vi "get_Image_from_multipage_TIFF.vi"(8 "error in (no error)":errorcluster, 11 "ImageCollection in":refnum<class "ImageCollection.lvclass">) -> (0 "error out":errorcluster, 2 "image":refnum<class "Image.lvclass">, 3 "ImageCollection out":refnum<class "ImageCollection.lvclass">)   [LabVIEW 2010]
uses:
  main/dlls/saveTiffStack_v02b/tiff_manage.dll
  Image/Image/Image.lvclass
  ImageCollection.lvclass
panel:
  in  "page_nr":u32=1
  out "return type":i32
  out "compression":u32
  out "bitspersample":u32
  out "length":u32
  out "width":u32
  out "status":u16
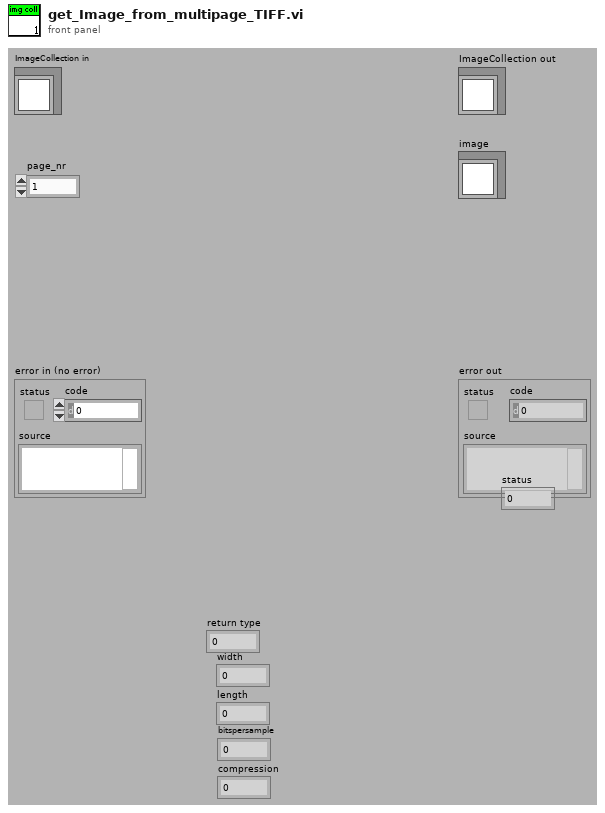
[diagram p1: front panel]
types:
  T1 = typedef "Image Type" = u32
  T2 = typedef "IMAQ Image.ctl" = refnum<image>
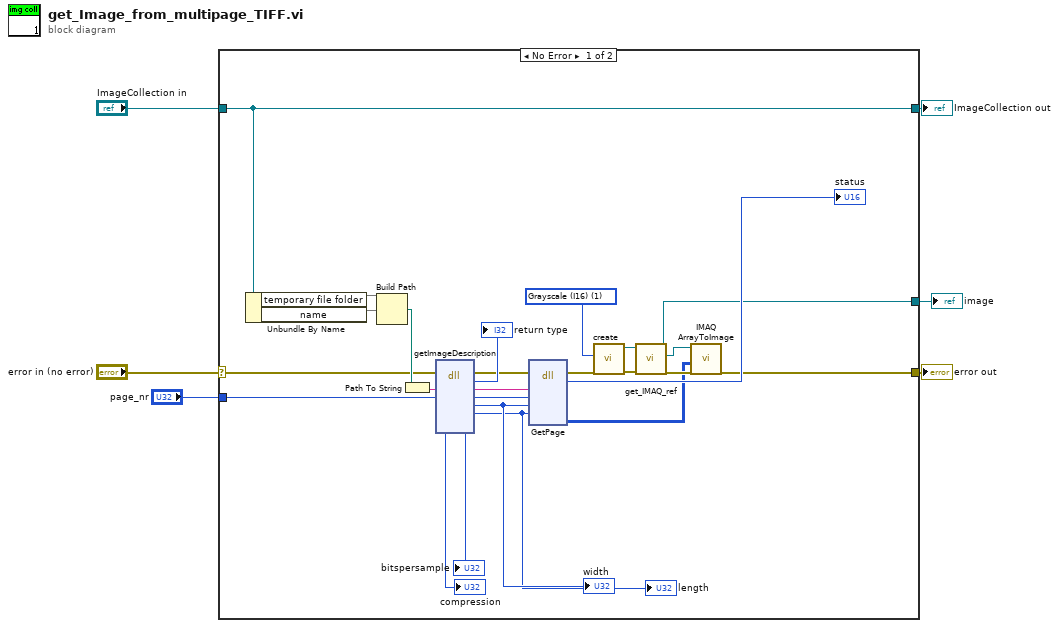
[diagram p0: block diagram]
diagram:
  n1 = case shown="No Error" "error in (no error)" {
    selector: "error in (no error)" -> [w19 w33]
    tunnel: [w13 w33] -> w5
    tunnel: [w31 w32] -> w3
    tunnel: "ImageCollection in" -> [w31 w32]
    tunnel: "page_nr" -> [w20 _]
    tunnel: [w9 _] -> w1
    frame No Error {
      w10 = T1 1 items=["Grayscale (U8)", "Grayscale (I16)", "Grayscale (SGL)", "Complex (CSG)", "RGB (U32)", "HSL (U32)", "RGB (U64)", "Grayscale (U16)"] ("Image Type")
      n2 = Unbundle By Name(w31) -> ("temporary file folder"=w30, "name"=w29)
      n3 = Build Path(base path=w30, name or relative path=w29) -> (appended path=w21:path)
      n4 = Path To String(path=w21) -> (string=w22:string)
      n5 = dll-call lib="C:/helioscan/main/dlls/saveTiffStack_v02b/tiff_manage.dll" fn="getImageDescription"(error in=w19, "path_filename"=w22, "page_nr"=w20) -> (error out=w18:errorcluster, "return value"=→"return type":i32, "path_filename"=w8:string, "page_nr"=w7:u32, "width"=w25:u32, "length"=w24:u32, "bitspersample"=→"bitspersample":u32, "compression"=→"compression":u32)  [unwired: 6 in, 1 out]
      "width" <- w25
      "length" <- w24
      n6 = dll-call lib="C:/helioscan/main/dlls/saveTiffStack_v02b/tiff_manage.dll" fn="GetPage"(error in=w18, "path_filename"=w8, "page_nr"=w7, "nrows"=w25, "ncols"=w24) -> (error out=w16:errorcluster, "return value"=→"status":u16, "in_array"=w12:u16[][])  [unwired: 7 in, 1 out]
      n7 = call "create.vi"("error in (no error)"=w16, "Image Type"=w10) -> ("error out"=w17:errorcluster, "Image out"=w15:refnum<class "Image.lvclass">)  [unwired: 8 in]
      n8 = call-dynamic "get_IMAQ_ref.vi"("error in (no error)"=w17, "Image.lvclass in"=w15) -> ("error out"=w14:errorcluster, "Image"=w11:T2, "Image.lvclass out"=w9:refnum<class "Image.lvclass">)  [unwired: 5 in, 2 out]
      n9 = call "IMAQ ArrayToImage"("error in (no error)"=w14, "Image Pixels (I16)"=w12, "Image"=w11) -> ("error out"=w13:errorcluster)  [unwired: 7 in, 1 out]
    }
    frame Error {
    }
  }
  "error out" <- w5
  "ImageCollection out" <- w3
  "image" <- w1
